vi "Send TX Message.vi"(8 "error in (no error)":errorcluster, 10 "element":string, 11 "RxTx in":refnum<class "RxTx.lvclass">) -> (0 "error out":errorcluster, 3 "RxTx out":refnum<class "RxTx.lvclass">)   [LabVIEW 2018, in "RxTx.lvclass"]
uses:
  RxTx.lvclass
  RxTx.lvclass/RxTx.ctl
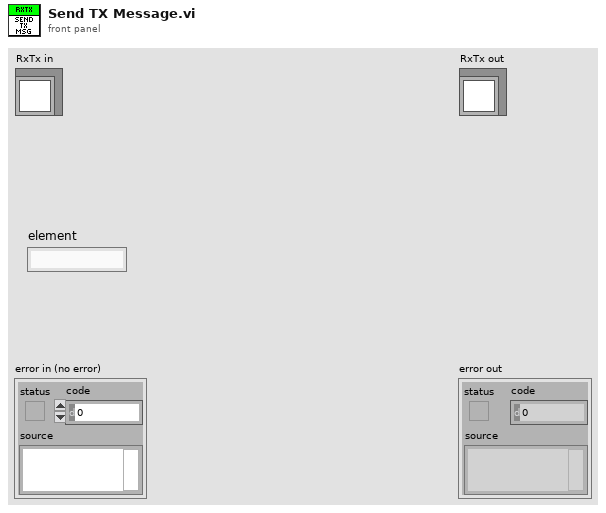
[diagram p1: front panel]
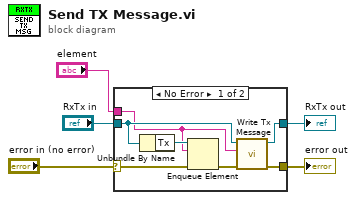
[diagram p0: block diagram]
diagram:
  n1 = case shown="No Error" "error in (no error)" {
    selector: "error in (no error)" -> [w11 w14]
    tunnel: [w9 w14] -> w4
    tunnel: [w7 w13] -> w2
    tunnel: "RxTx in" -> [w8 w13]
    tunnel: "element" -> [w6 _]
    frame No Error {
      n2 = Unbundle By Name(w8) -> ("Tx"=w12:refnum<queue>)
      n3 = Enqueue Element(queue=w12, element=w6, error in (no error)=w11) -> (error out=w10:errorcluster)  [unwired: 1 in, 2 out]
      n4 = call "Write Tx Message.vi"("error in (no error)"=w10, "Tx Message"=w6, "RxTx in"=w8) -> ("error out"=w9:errorcluster, "RxTx out"=w7:refnum<class "RxTx.lvclass">)  [unwired: 7 in]
    }
    frame Error {
    }
  }
  "error out" <- w4
  "RxTx out" <- w2
